vi "E2 Data Logger.vi"(7 "refnum in":refnum<file>) -> (3 "refnum out":refnum<file>)   [LabVIEW 2015]
uses:
  <vilib>/Rock Robotics/WPI/DriverStation/WPI_DriverStationRobotMode2.ctl
  Robot Global Data.vi
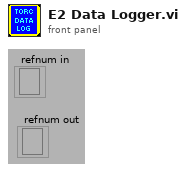
[diagram p1: front panel]
types:
  T1 = typedef "WPI_DriverStationRobotMode2.ctl" = enum16{"Autonomous Disabled", "Autonomous Enabled", "Teleop Disabled", "Teleop Enabled", "Disconnected", "Finish", "Test Disabled", "Test Enabled", "Emergency Stopped"}
  T2 = enum16{"CW_Fast", "CW_Slow", "CCW_Fast", "CCW_Slow", "Straight", "WaitingForStraight", "Rotate_Move"}
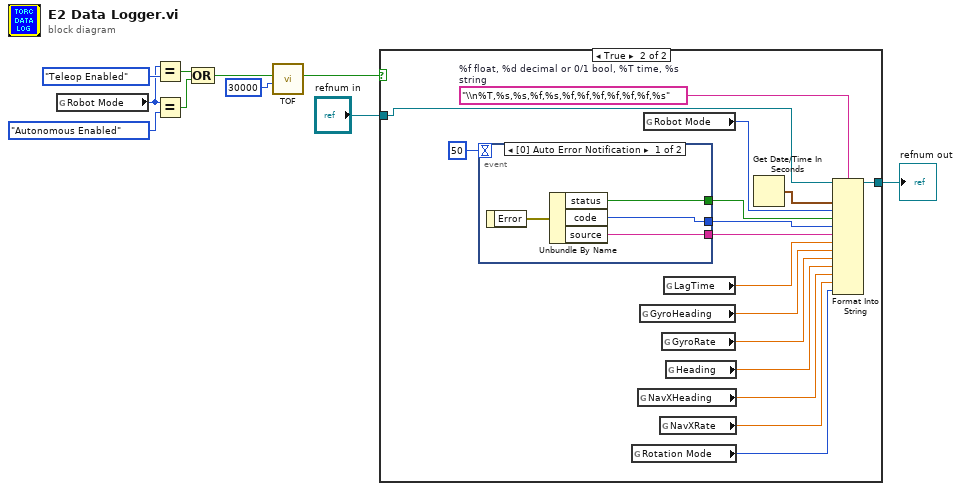
[diagram p0: block diagram]
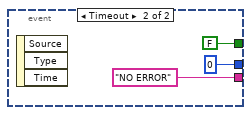
[diagram p3: hidden frame]
diagram:
  n1 = global read "Robot Global Data.vi" "Robot Mode"() -> (w4:T1)
  n2 = Equal?(x=w4, y=WPI_DriverStationRobotMode2."Teleop Enabled") -> (x = y?=w6:bool)
  n3 = Equal?(x=w4, y=WPI_DriverStationRobotMode2."Autonomous Enabled") -> (x = y?=w5:bool)
  n4 = Compound Arithmetic op=OR(w6, w5) -> (w3:bool)
  n5 = call "TOF.vi"("Delay (ms)"=u32 30000, "Input"=w3) -> ("Output"=w2:bool)  [unwired: 9 in]
  n6 = case shown="True" w2 {
    tunnel: [w11 w27] -> w10
    tunnel: "refnum in" -> [w11 w23]
    frame False {
    }
    frame True {
      w24 = "\\n%T,%s,%s,%f,%s,%f,%f,%f,%f,%f,%f,%s"  # %f float, %d decimal or 0/1 bool, %T time, %s string
      n7 = event shown="[0] Auto Error Notification" {
        selector: _ -> [_ _]
        dyn-events: _ -> [_ _]
        timeout: 50 -> [_ _]
        tunnel: [w30 "NO ERROR" ("source")] -> w19
        tunnel: [w29 0 ("code")] -> w20
        tunnel: [w28 FALSE ("status")] -> w21
        event Auto Error Notification {
          n8 = event-data() -> ("Error"=w31:errorcluster)  [unwired: 1 in]
          n9 = Unbundle By Name(w31) -> ("status"=w28:bool, "code"=w29:i32, "source"=w30:string)
        }
        event Timeout {
          n10 = event-data() -> ()  [unwired: 1 in, 3 out]
        }
      }
      n11 = global read "Robot Global Data.vi" "Rotation Mode"() -> (w12:T2)
      n12 = global read "Robot Global Data.vi" "NavXHeading"() -> (w14:dbl)
      n13 = global read "Robot Global Data.vi" "GyroHeading"() -> (w17:dbl)
      n14 = global read "Robot Global Data.vi" "Robot Mode"() -> (w25:T1)
      n15 = global read "Robot Global Data.vi" "NavXRate"() -> (w13:dbl)
      n16 = global read "Robot Global Data.vi" "GyroRate"() -> (w16:dbl)
      n17 = global read "Robot Global Data.vi" "LagTime"() -> (w18:dbl)
      n18 = global read "Robot Global Data.vi" "Heading"() -> (w15:dbl)
      n19 = Get Date/Time In Seconds() -> (seconds since 1Jan1904=w26:timestamp)
      n20 = Format Into String(format string=w24, initial string=w23, w26, w25, w21, w20, w19, w18, w17, w16, w15, w14, w13, w12) -> (resulting string=w27:refnum<file>)  [unwired: 1 in, 1 out]
    }
  }
  "refnum out" <- w10
